vi "MKS CTLR - Error Handler.vi"(8 "error in (no error)":errorcluster, 11 "VISA resource name (IN)":refnum<visa-resource-name>) -> (0 "error out":errorcluster, 3 "VISA resource name (OUT)":refnum<visa-resource-name>)   [LabVIEW 2013]
uses:
  <vilib>/Utility/error.llb/DialogType.ctl
  Global - Pressure & Flow.vi
panel:
  out "Time Stamp":timestamp
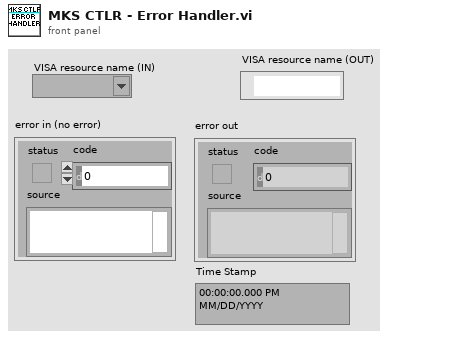
[diagram p1: front panel]
types:
  T1 = typedef "DialogType.ctl" = u16
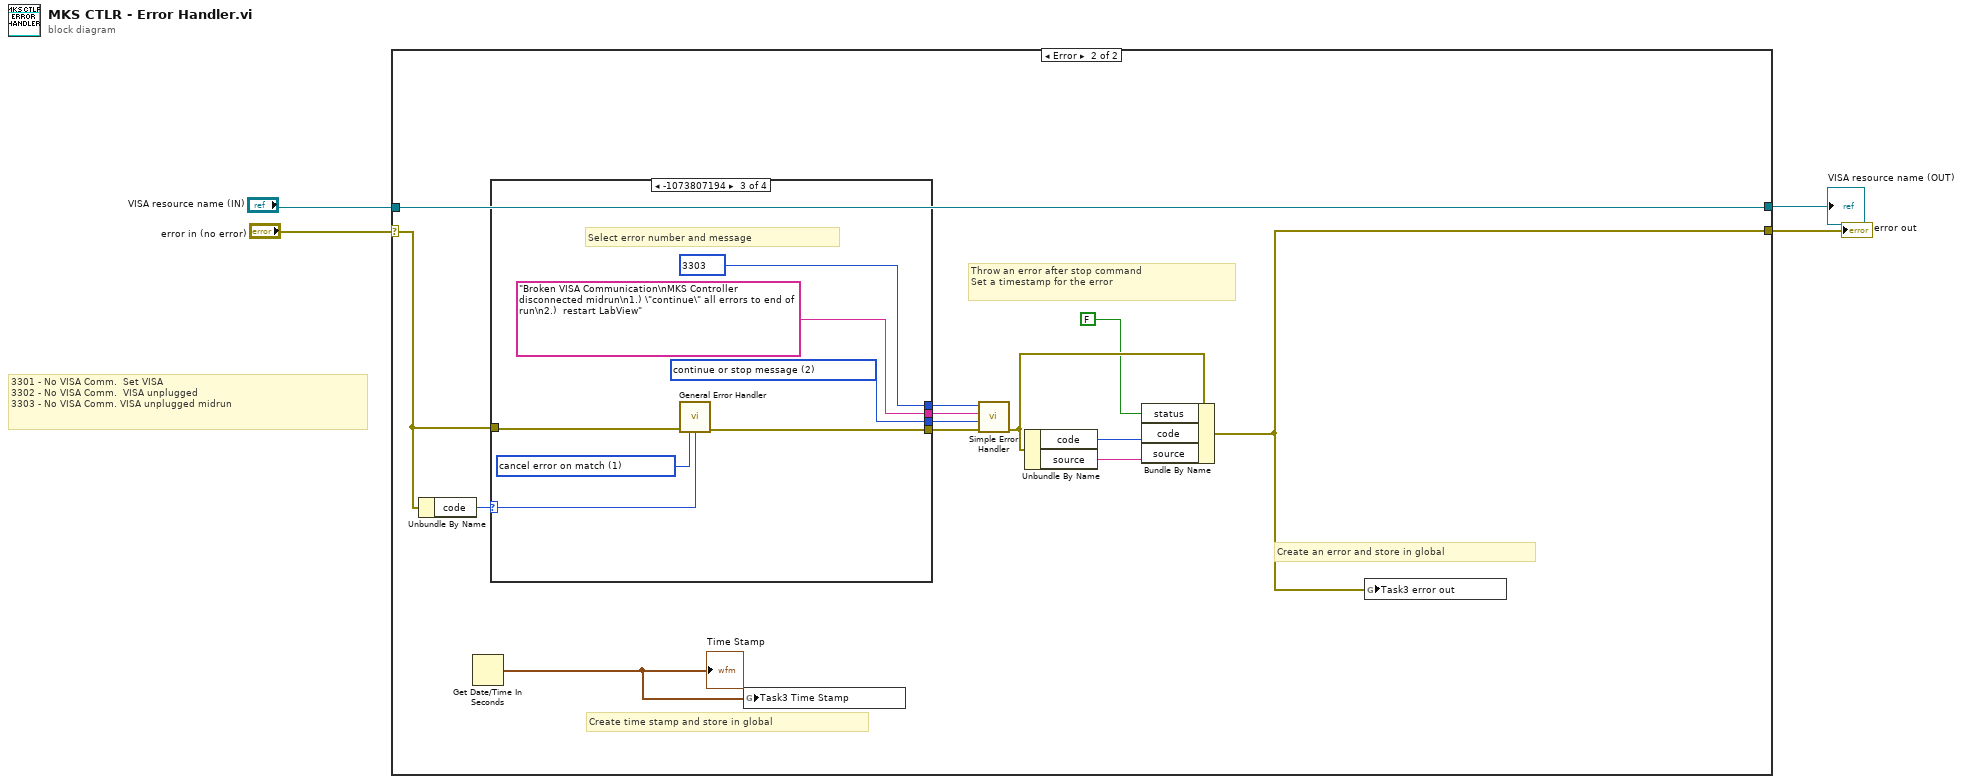
[diagram p0: block diagram]
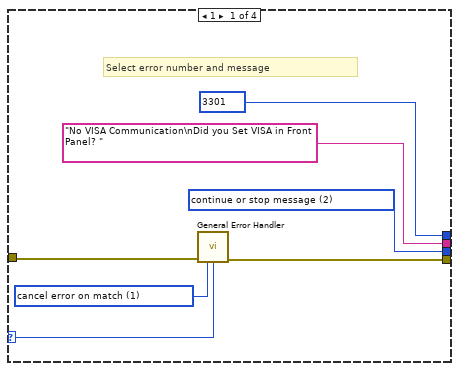
[diagram p3: hidden frame]
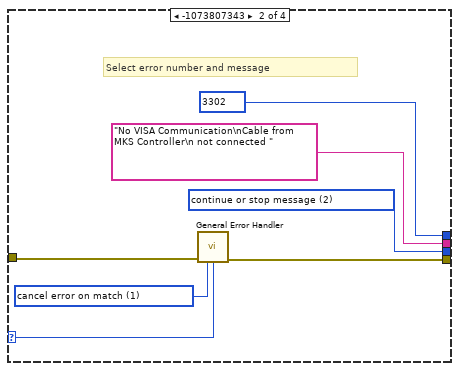
[diagram p4: hidden frame]
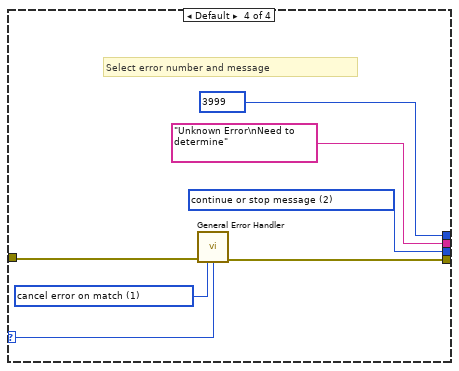
[diagram p5: hidden frame]
diagram:
  # "3301 - No VISA Comm.  Set VISA\n3302 - No VISA Comm.  VISA unplugged\n3303 - No VISA Comm. VISA unplugged midrun"
  n1 = case shown="Error" "error in (no error)" {
    selector: "error in (no error)" -> [w6 w7]
    tunnel: "VISA resource name (IN)" -> [w5 w9]
    tunnel: [w6 w12] -> w3
    tunnel: [w5 w9] -> w1
    frame No Error {
    }
    frame Error {
      # "Create time stamp and store in global"
      # "Throw an error after stop command\nSet a timestamp for the error"
      # "Create an error and store in global"
      n2 = Unbundle By Name(w7) -> ("code"=w8:i32)
      n3 = Get Date/Time In Seconds() -> (seconds since 1Jan1904=w18:timestamp)
      "Time Stamp" <- w18
      n4 = case shown="-1073807194" w8 {
        selector: w8 -> [w21 w28 w35 w42]
        tunnel: [w26 w33 w40 w47] -> w19
        tunnel: ["No VISA Communication\nDid you Set VISA in Front Panel? " ("[error source] (\" \")") "No VISA Communication\nCable from MKS Controller\n not connected " ("[error source] (\" \")") "Broken VISA Communication\nMKS Controller disconnected midrun\n1.) \"continue\" all errors to end of run\n2.)  restart LabView" ("[error source] (\" \")") "Unknown Error\nNeed to determine" ("[error source] (\" \")")] -> w14
        tunnel: [3301 ("[error code] (0)") 3302 ("[error code] (0)") 3303 ("[error code] (0)") 3999 ("[error code] (0)")] -> w13
        tunnel: [w22 w29 w36 w43] -> w10
        tunnel: w7 -> [w20 w27 w34 w41]
        frame 1 {
          w23 = 1 items=["no exception", "cancel error on match", "set error on match"] ("[exception action] (none:0)")
          w26 = T1 2 items=["no dialog", "OK message", "continue or stop message", "OK message + warnings", "continue/stop + warnings"] ("type of dialog (OK msg:1)")
          # "Select error number and message"
          n5 = call <vilib>:"General Error Handler.vi"("error in (no error)"=w20, "[exception action] (none:0)"=w23, "[exception code]"=w21) -> ("error out"=w22:errorcluster)  [unwired: 8 in, 4 out]
        }
        frame -1073807343 {
          w30 = 1 items=["no exception", "cancel error on match", "set error on match"] ("[exception action] (none:0)")
          w33 = T1 2 items=["no dialog", "OK message", "continue or stop message", "OK message + warnings", "continue/stop + warnings"] ("type of dialog (OK msg:1)")
          # "Select error number and message"
          n6 = call <vilib>:"General Error Handler.vi"("error in (no error)"=w27, "[exception action] (none:0)"=w30, "[exception code]"=w28) -> ("error out"=w29:errorcluster)  [unwired: 8 in, 4 out]
        }
        frame -1073807194 {
          w37 = 1 items=["no exception", "cancel error on match", "set error on match"] ("[exception action] (none:0)")
          w40 = T1 2 items=["no dialog", "OK message", "continue or stop message", "OK message + warnings", "continue/stop + warnings"] ("type of dialog (OK msg:1)")
          # "Select error number and message"
          n7 = call <vilib>:"General Error Handler.vi"("error in (no error)"=w34, "[exception action] (none:0)"=w37, "[exception code]"=w35) -> ("error out"=w36:errorcluster)  [unwired: 8 in, 4 out]
        }
        frame Default {
          w44 = 1 items=["no exception", "cancel error on match", "set error on match"] ("[exception action] (none:0)")
          w47 = T1 2 items=["no dialog", "OK message", "continue or stop message", "OK message + warnings", "continue/stop + warnings"] ("type of dialog (OK msg:1)")
          # "Select error number and message"
          n8 = call <vilib>:"General Error Handler.vi"("error in (no error)"=w41, "[exception action] (none:0)"=w44, "[exception code]"=w42) -> ("error out"=w43:errorcluster)  [unwired: 8 in, 4 out]
        }
      }
      n9 = global write "Global - Pressure & Flow.vi" "Task3 Time Stamp"(w18) -> ()
      n10 = call <vilib>:"Simple Error Handler.vi"("error code (no error:0)"=w13, "error source (\" \")"=w14, "type of dialog (OK msg:1)"=w19, "error in (no error)"=w10) -> ("error out"=w15:errorcluster)  [unwired: 1 in, 4 out]
      n11 = Unbundle By Name(w15) -> ("code"=w17:i32, "source"=w16:string)
      n12 = Bundle By Name(cluster=w15, "status"=FALSE, "code"=w17, "source"=w16) -> (w12:errorcluster)
      n13 = global write "Global - Pressure & Flow.vi" "Task3 error out"(w12) -> ()
    }
  }
  "error out" <- w3
  "VISA resource name (OUT)" <- w1
